vi "AIDI-Initialize AI.vi"(0 "AI":T2, 7 "external trig":bool, 9 "Sync task in":refnum<k21>, 11 "error in (no error)":errorcluster) -> (4 "Tasks Out":T1[](array[typedef]), 8 "order":i32[](array[numeric]), 10 "Sync task out":refnum<k21>, 15 "error out":errorcluster)   [LabVIEW 2020]
uses:
  Typedefs/AIDI-Output Spec.ctl
  Typedefs/AIDI-Task Specification.ctl
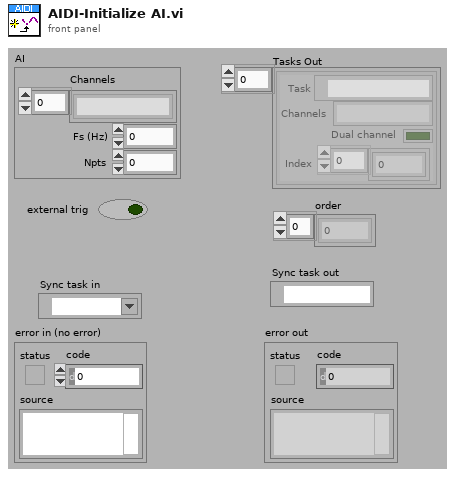
[diagram p1: front panel]
types:
  T1 = typedef "AIDI-Task Specification.ctl" = cluster{"Task":refnum<k21>, "Channels":string, "Dual channel":bool, "Index":i32[]}
  T2 = typedef "AIDI-Output Spec.ctl" = cluster{"Channels":string[], "Fs (Hz)":dbl, "Npts":i32}
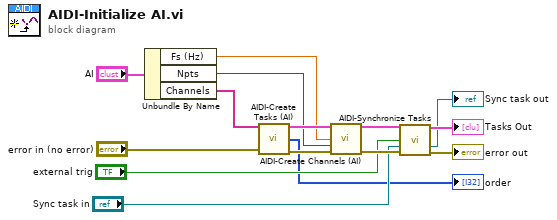
[diagram p0: block diagram]
diagram:
  n1 = Unbundle By Name("AI") -> ("Fs (Hz)"=w11:dbl, "Npts"=w5:i32, "Channels"=w6:string[])
  n2 = call "AIDI-Create Tasks (AI).vi"("Channels"=w6, "error in (no error)"="error in (no error)") -> ("Task Specs"=w13:T1[], "order"=→"order":i32[], "error out"=w12:errorcluster)  [unwired: 11 in]
  n3 = call "AIDI-Create Channels (AI).vi"("Tasks In"=w13, "Fs (Hz)"=w11, "Npts"=w5, "error in (no error)"=w12) -> ("Tasks Out"=w10:T1[], "error out"=w9:errorcluster)  [unwired: 10 in]
  n4 = call "AIDI-Synchronize Tasks.vi"("Tasks In"=w10, "external trig"="external trig", "Sync task in"="Sync task in", "error in (no error)"=w9) -> ("Tasks Out"=→"Tasks Out":T1[], "Sync task out"=→"Sync task out":refnum<k21>, "error out"=→"error out":errorcluster)  [unwired: 9 in]
